vi "AddonMotor Speed.vi"(6 "Duration":dbl=50.0, 7 "Description":string="Reserve", 8 "Command Info In":T1, 10 "Speed":dbl, 11 "Motor ID":dbl) -> (0 "Command Info":T1)   [LabVIEW 2015]
uses:
  <vilib>/Rock Robotics/WPI/Framework/Command Status Info.ctl
  <vilib>/Rock Robotics/WPI/Framework/Completion Status.ctl
  <vilib>/Rock Robotics/WPI/Framework/Completion Notifier.ctl
  Implementation/AddonMotors Setpoints.ctl
  Implementation/AddonMotors Operations.ctl
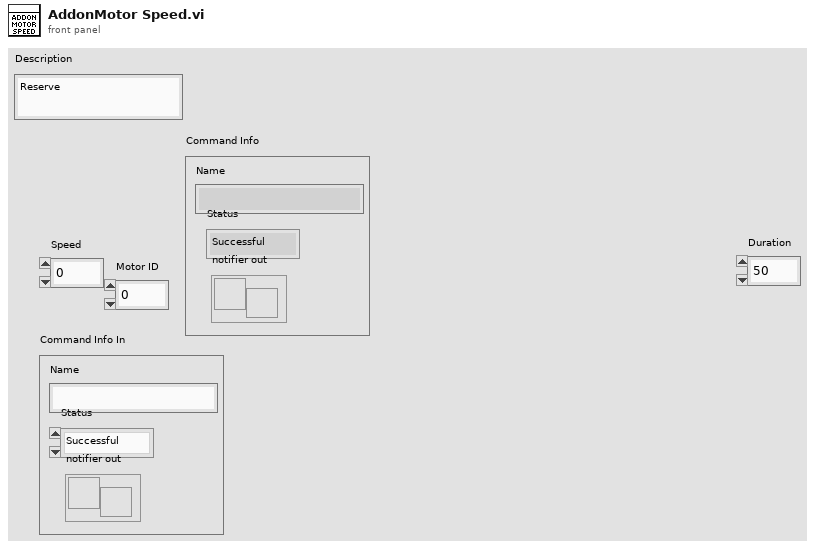
[diagram p1: front panel]
types:
  T1 = typedef "Command Status Info.ctl" = cluster{"Name":string, "Status":T2, "notifier out":T3}
  T2 = typedef "Completion Status.ctl" = enum16{"Successful", "Aborted", "Incomplete"}
  T3 = typedef "Completion Notifier.ctl" = refnum<notifier>
  T4 = typedef "AddonMotors Setpoints.ctl" = cluster{"Operation":T5, "Setpoint":dbl, "Duration":dbl, "Motor ID":dbl}
  T5 = typedef "AddonMotors Operations.ctl" = enum16{"Reserve", "Read Current", "Immediate", "Angle (Position)", "Speed", "Angle Increments (Position)"}
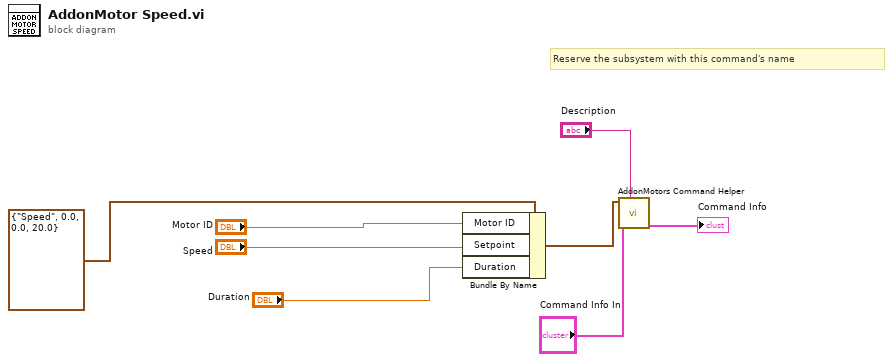
[diagram p0: block diagram]
diagram:
  # "Reserve the subsystem with this command's name"
  n1 = Bundle By Name(cluster=T4 {"Operation"=enum."Speed", "Setpoint"=0.0, "Duration"=0.0, "Motor ID"=20.0} ("SubSystem Data"), "Motor ID"="Motor ID", "Setpoint"="Speed", "Duration"="Duration") -> (w5:T4)
  n2 = call "AddonMotors Command Helper.vi"("Description"="Description", "Command Info In"="Command Info In", "SubSystem Data"=w5) -> ("Command Info Out"=→"Command Info":T1)  [unwired: 7 in, 1 out]
